vi "instantiate_embed_nodes.vi"(0 "abstract_llm_embedding":refnum<class "abstract_llm_base.lvclass">, 11 "error in (no error)":errorcluster) -> (4 "embed_nodes out":refnum<class "embed_nodes.lvclass">, 15 "error out":errorcluster)   [LabVIEW 2020, in "embed_nodes.lvclass"]
uses:
  embed_nodes.lvclass
  models/abstract_llm_base/abstract_llm_base.lvclass
  embed_nodes.lvclass/embed_nodes.ctl
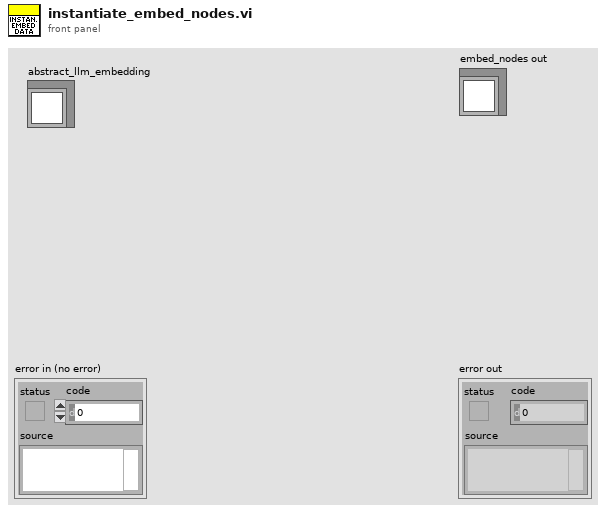
[diagram p1: front panel]
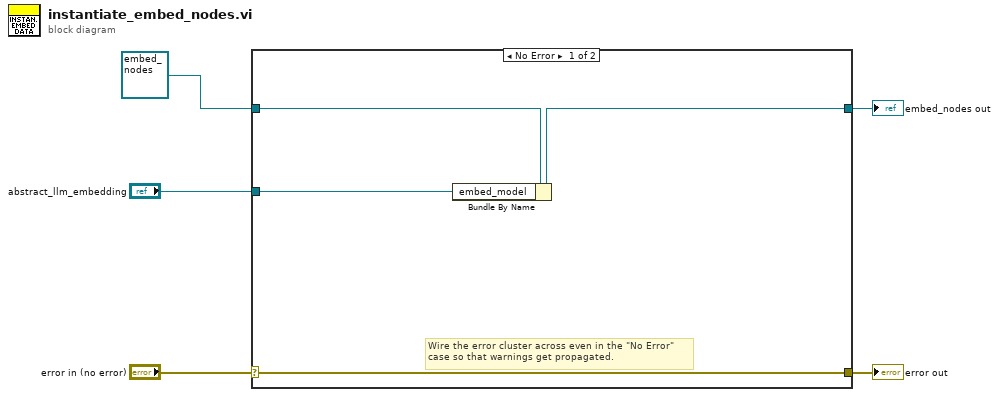
[diagram p0: block diagram]
diagram:
  n1 = case shown="No Error" "error in (no error)" {
    selector: "error in (no error)" -> [w9 w11]
    tunnel: [w9 w11] -> w4
    tunnel: [w6 w10] -> w2
    tunnel: refnum<class "embed_nodes.lvclass"> refnum ("embed_nodes in") -> [w8 w10]
    tunnel: "abstract_llm_embedding" -> [w7 _]
    frame No Error {
      # "Wire the error cluster across even in the \"No Error\"\ncase so that warnings get propagated."
      n2 = Bundle By Name(cluster=w8, "embed_model"=w7) -> (w6:refnum<class "embed_nodes.lvclass">)
    }
    frame Error {
    }
  }
  "error out" <- w4
  "embed_nodes out" <- w2
